vi "ScanDurationEstimator2.vi"(1 "#points":i32, 2 "charge":bool, 3 "Time [s]":dbl) -> (0 "concatenated string":string)   [LabVIEW 2015]
panel:
  out "Min":string
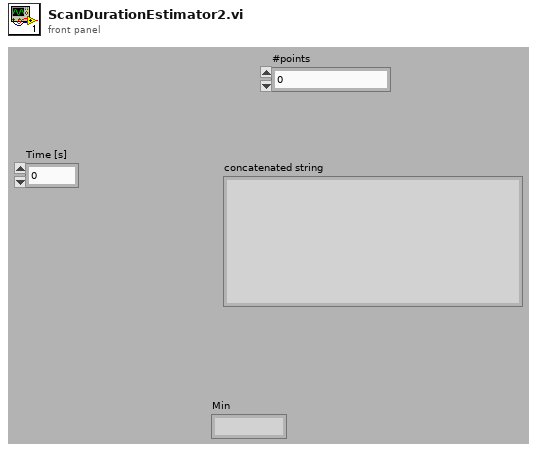
[diagram p1: front panel]
types:
  T1 = typedef "LVDateTimeRec.ctl" = cluster{"fractional second":dbl, "second":i32, "minute":i32, "hour":i32, "day of month":i32, "month":i32, "year":i32, "day of week":i32, "day of year":i32, "DST":i32}
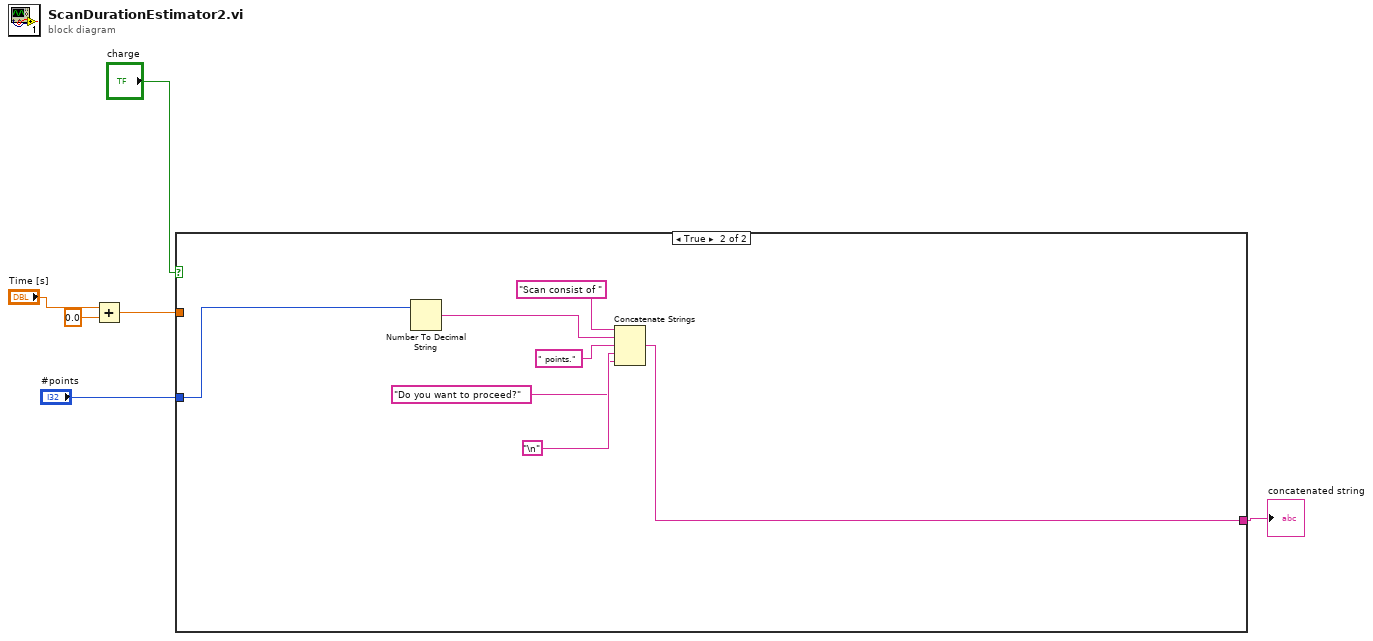
[diagram p0: block diagram]
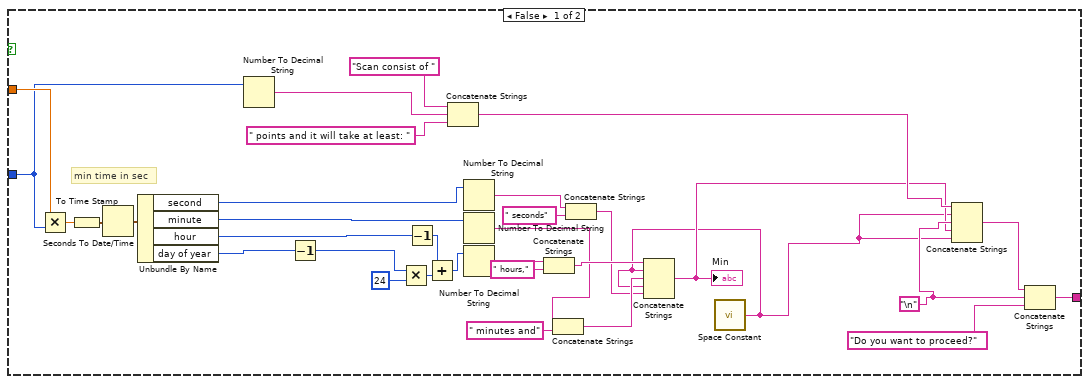
[diagram p2: hidden frame]
diagram:
  n1 = Add(x="Time [s]", y=0.0) -> (x+y=w4:dbl)
  n2 = case shown="True" "charge" {
    tunnel: w4 -> [w39 _]
    tunnel: [w27 w40] -> w3
    tunnel: "#points" -> [w24 w46]
    frame False {
      w19 = "\n"
      # "min time in sec"
      n3 = Multiply(x=w39, y=w24) -> (x*y=w32:dbl)
      n4 = To Time Stamp(1:w32) -> (0:w37:timestamp)
      n5 = Seconds To Date/Time(time stamp (now)=w37) -> (date time rec=w38:T1)  [unwired: 1 in]
      n6 = Unbundle By Name(w38) -> ("second"=w31:i32, "minute"=w30:i32, "hour"=w29:i32, "day of year"=w26:i32)
      n7 = Number To Decimal String(number=w24) -> (decimal integer string=w22:string)  [unwired: 1 in]
      n8 = Decrement(x=w26) -> (x-1=w25:i32)
      n9 = Multiply(x=w25, y=24) -> (x*y=w33:i32)
      n10 = Decrement(x=w29) -> (x-1=w35:i32)
      n11 = Add(x=w35, y=w33) -> (x+y=w34:i32)
      n12 = Concatenate Strings("Scan consist of " ("string"), w22, " points and it will take at least: " ("string")) -> (w20:string)
      n13 = Number To Decimal String(number=w31) -> (decimal integer string=w10:string)  [unwired: 1 in]
      n14 = Number To Decimal String(number=w30) -> (decimal integer string=w13:string)  [unwired: 1 in]
      n15 = Number To Decimal String(number=w34) -> (decimal integer string=w17:string)  [unwired: 1 in]
      n16 = Concatenate Strings(w17, " hours," ("string")) -> (w15:string)
      n17 = Concatenate Strings(w13, " minutes and" ("string")) -> (w12:string)
      n18 = Concatenate Strings(w10, " seconds" ("string")) -> (w9:string)
      n19 = call <vilib>:"Space Constant.vi"() -> ("String"=w7:string)
      n20 = Concatenate Strings(w15, w7, w12, w7, w9) -> (w18:string)
      "Min" <- w18
      n21 = Concatenate Strings(w20, w7, w19, w18, w7) -> (w28:string)
      n22 = Concatenate Strings(w28, w19, "Do you want to proceed?" ("string")) -> (w27:string)
    }
    frame True {
      n23 = Number To Decimal String(number=w46) -> (decimal integer string=w44:string)  [unwired: 1 in]
      n24 = Concatenate Strings("Scan consist of " ("string"), w44, " points." ("string"), "\n", "Do you want to proceed?" ("string")) -> (w40:string)
    }
  }
  "concatenated string" <- w3
